vi "Write Data.vi"(6 "Time End":timestamp, 7 "Time Start":timestamp, 8 "error in":errorcluster, 9 "Success?":bool, 10 "Project Action":refnum<class "Project Action.lvclass">, 11 "Report Data in":refnum<class "Report Data.lvclass">) -> (0 "error dub":errorcluster, 3 "Report Data out":refnum<class "Report Data.lvclass">)   [LabVIEW 2019, in "ProjectBuilder.lvlib" / "Report Data.lvclass"]
doc: "Write data."
uses:
  Report Data.lvclass
  Project Action/Project Action.lvclass
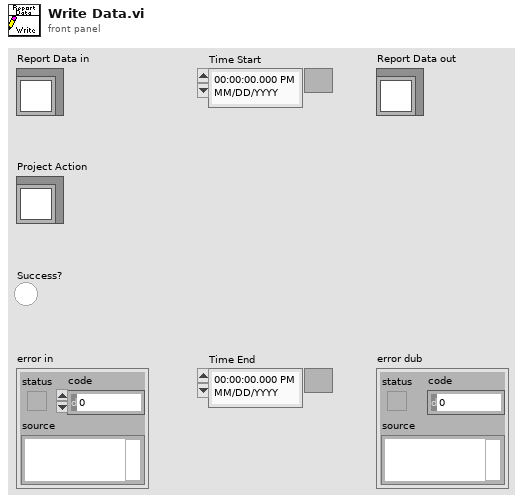
[diagram p1: front panel]
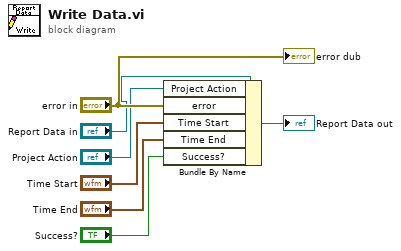
[diagram p0: block diagram]
diagram:
  n1 = Bundle By Name(cluster="Report Data in", "Project Action"="Project Action", "error"="error in", "Time Start"="Time Start", "Time End"="Time End", "Success?"="Success?") -> (→"Report Data out":refnum<class "Report Data.lvclass">)
  "error dub" <- "error in"
